vi "Waveform - Scale and Offset.vi"() -> ()   [LabVIEW 2023]
doc: "Shows how to multiply the waveform by a scalar factor and add an offset."
panel:
  in  "Scale":dbl=4.0
  in  "Offset":dbl=50.0
  out "Waveform Graph":waveform(dbl)[](graph)
  # "Overview: Demonstrates how to apply a scale and an offset to an existing waveform with the Waveform Scale and Offset VI.\nInstructions:\n1. Specify Scale and Offset values.\n2. Run the VI. The scaled data will display the result of applying the scale and offset to the original data."
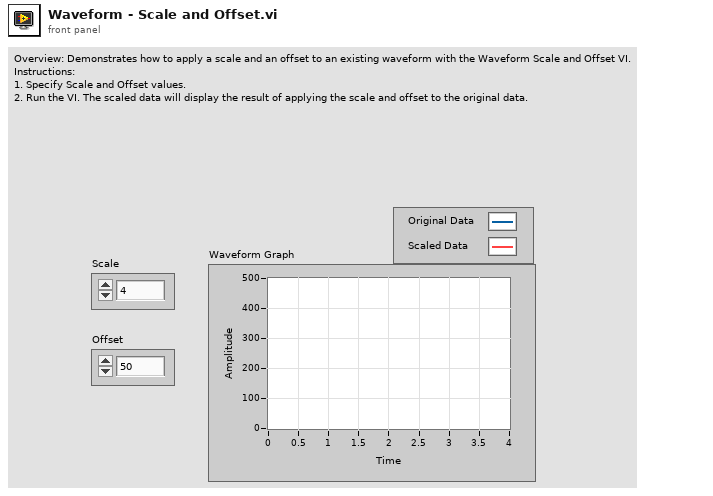
[diagram p1: front panel]
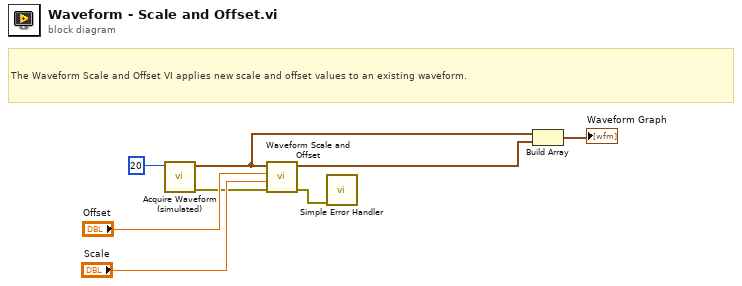
[diagram p0: block diagram]
diagram:
  # "The Waveform Scale and Offset VI applies new scale and offset values to an existing waveform."
  n1 = call "Acquire Waveform (simulated).vi"("# points"=20) -> ("error out"=w1:errorcluster, "waveform output"=w7:waveform(dbl))  [unwired: 9 in]
  n2 = call <vilib>:"Waveform Scale and Offset.vi"("error in (no error)"=w1, "scale"="Scale", "offset"="Offset", "waveform in"=w7) -> ("error out"=w2:errorcluster, "waveform out"=w4:waveform(dbl))  [unwired: 6 in]
  n3 = call <vilib>:"Simple Error Handler.vi"("error in (no error)"=w2) -> ()  [unwired: 4 in, 5 out]
  n4 = Build Array(w7, w4) -> (→"Waveform Graph":waveform(dbl)[])
